vi "Description_parameter_type_float_unicorn_(SubVI).vi"(10 "Numeric":i32, 11 "Param":T1) -> (3 "ParamFloat":T2)   [LabVIEW 2017, in "LV_Unicorn.lvlib"]
uses:
  LV_Unicorn.lvlib
  Control/unicorn_DescriptParam.ctl
  Control/unicorn_ParamFloat.ctl
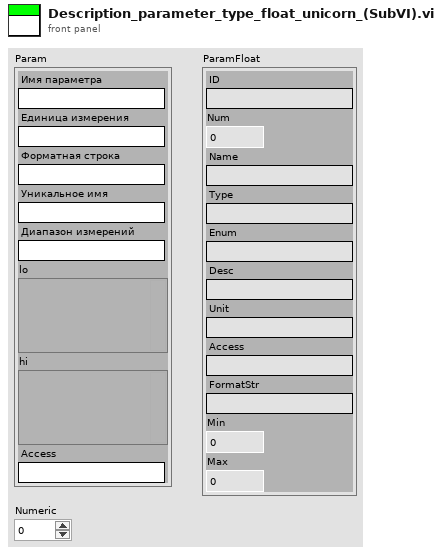
[diagram p1: front panel]
types:
  T1 = typedef "unicorn_DescriptParam.ctl" = cluster{"Имя параметра":string, "Единица измерения":string, "Форматная строка ":string, "Уникальное имя":string, "Диапазон измерений":string, "lo":variant, "hi":variant, "Access":string}
  T2 = cluster{"ID":string, "Num":i32, "Name":string, "Type":string, "Enum":string, "Desc":string, "Unit":string, "Access":string, "FormatStr":string, "Min":i32, "Max":i32}
  T3 = typedef "LV_Unicorn.lvlib/unicorn_ParamFloat.ctl" = cluster{"ID":string, "Num":i32, "Name":string, "Type":string, "Enum":string, "Desc":string, "Unit":string, "Access":string, "FormatStr":string, "Min":sgl, "Max":sgl}[]
  T4 = cluster{"ID":string, "Num":i32, "Name":string, "Type":string, "Enum":string, "Desc":string, "Unit":string, "Access":string, "FormatStr":string, "Min":sgl, "Max":sgl}
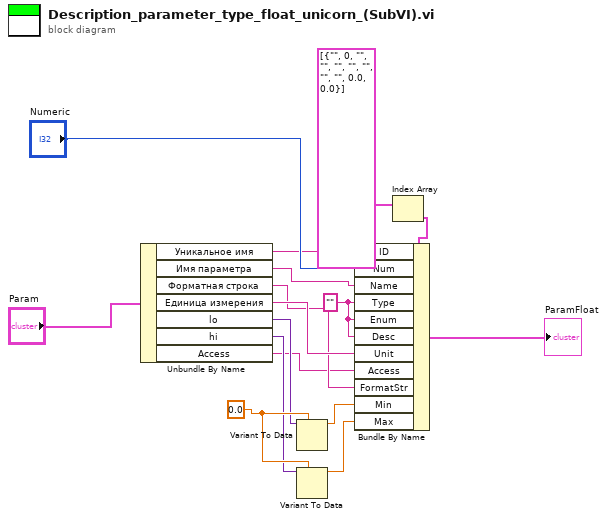
[diagram p0: block diagram]
diagram:
  w16 = "" ("Type")
  w12 = sgl 0.0 ("Min")
  n1 = Unbundle By Name("Param") -> ("Уникальное имя"=w4:string, "Имя параметра"=w6:string, "Форматная строка"=w14:string, "Единица измерения"=w15:string, "lo"=w9:variant, "hi"=w11:variant, "Access"=w8:string)
  n2 = Variant To Data(type=w12, Variant=w9) -> (data=w10:sgl)  [unwired: 1 in, 1 out]
  n3 = Variant To Data(type=w12, Variant=w11) -> (data=w13:sgl)  [unwired: 1 in, 1 out]
  n4 = Index Array(array=T3 [{"ID"="", "Num"=0, "Name"="", "Type"="", "Enum"="", "Desc"="", "Unit"="", "Access"="", "FormatStr"="", "Min"=0.0, "Max"=0.0}] ("ParamInt 2")) -> (element=w2:T4)  [unwired: 1 in]
  n5 = Bundle By Name(cluster=w2, "ID"=w4, "Num"="Numeric", "Name"=w6, "Type"=w16, "Enum"=w16, "Desc"=w16, "Unit"=w15, "Access"=w8, "FormatStr"=w14, "Min"=w10, "Max"=w13) -> (→"ParamFloat":T4)
